vi "GitCheckRepo.vi"(8 "error in (no error)":errorcluster, 9 "Directory":path=path "", 11 "Git exec":string="git") -> (0 "error out":errorcluster, 1 "Directory out":path, 2 "ProcedureRepo?":bool, 3 "Git exec out":string="git")   [LabVIEW 2013]
uses:
  GitInterface/GitCmd.vi
  <vilib>/dlg_ctls.llb/Space Constant.vi
  PathtoDirPath.vi
  <vilib>/Platform/system.llb/System Exec.vi
  <vilib>/Utility/error.llb/Error Cluster From Error Code.vi
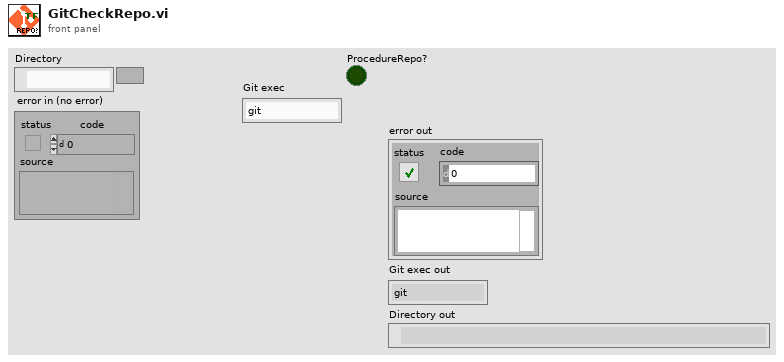
[diagram p1: front panel]
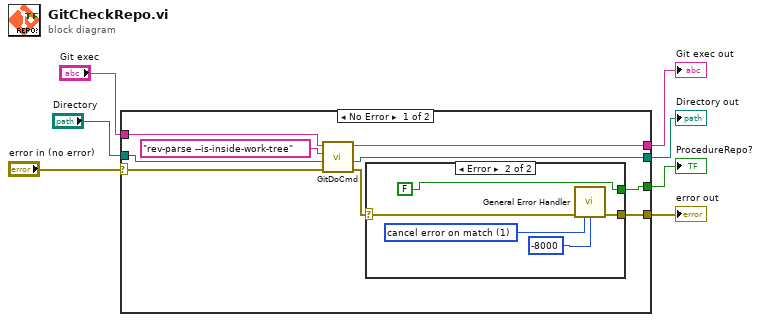
[diagram p0: block diagram]
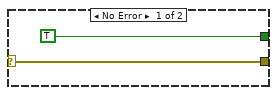
[diagram p2: hidden frame]
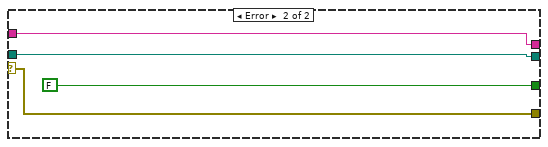
[diagram p3: hidden frame]
diagram:
  n1 = case shown="No Error" "error in (no error)" {
    selector: "error in (no error)" -> [w16 w27]
    tunnel: "Git exec" -> [w14 w25]
    tunnel: "Directory" -> [w15 w26]
    tunnel: [w11 FALSE ("selection")] -> w1
    tunnel: [w8 w27] -> w5
    tunnel: [w12 w26] -> w3
    tunnel: [w10 w25] -> w2
    frame No Error {
      n2 = call "GitDoCmd.vi"("error in (no error)"=w16, "Working Path"=w15, "Git command"="rev-parse --is-inside-work-tree" ("string"), "Git exec"=w14) -> ("error out"=w9:errorcluster, "Working Path out"=w12:path, "Git exec out"=w10:string)  [unwired: 3 in, 1 out]
      n3 = case shown="Error" w9 {
        selector: w9 -> [w18 w21]
        tunnel: [TRUE ("selection") FALSE ("selection")] -> w11
        tunnel: [w18 w20] -> w8
        frame No Error {
        }
        frame Error {
          w22 = 1 items=["no exception", "cancel error on match", "set error on match"] ("[exception action] (none:0)")
          n4 = call <vilib>:"General Error Handler.vi"("error in (no error)"=w21, "[exception action] (none:0)"=w22, "[exception code]"=-8000) -> ("error out"=w20:errorcluster)  [unwired: 8 in, 4 out]
        }
      }
    }
    frame Error {
    }
  }
  "error out" <- w5
  "Git exec out" <- w2
  "Directory out" <- w3
  "ProcedureRepo?" <- w1
